vi "niRFUtil CONV 1 Ohm Voltage to dBm (complex scalar).vi"(7 "Complex Scalar (V)":csg format="%.2f") -> (8 "Real Scalar (dBm)":sgl format="%.2f")   [LabVIEW 2015, in "niRFUtil.lvlib"]
doc: "(c) Copyright 2006, National Instruments, Inc. This VI may not be duplicated, sold, or distributed without written consent from National Instruments."
uses:
  niRFUtil.lvlib
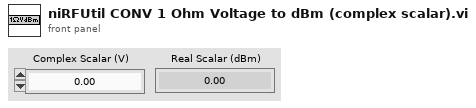
[diagram p1: front panel]
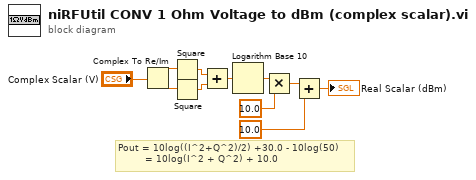
[diagram p0: block diagram]
diagram:
  # "Pout = 10log((I^2+Q^2)/2) +30.0 - 10log(50)\n         = 10log(I^2 + Q^2) + 10.0"
  n1 = Complex To Re/Im(x + iy="Complex Scalar (V)") -> (x=w7:sgl, y=w6:sgl)
  n2 = Square(x=w7) -> (x^2=w5:sgl)
  n3 = Square(x=w6) -> (x^2=w4:sgl)
  n4 = Add(x=w5, y=w4) -> (x+y=w3:sgl)
  n5 = Logarithm Base 10(1:w3) -> (0:w11:sgl)
  n6 = Multiply(x=w11, y=sgl 10.0) -> (x*y=w9:sgl)
  n7 = Add(x=w9, y=sgl 10.0) -> (x+y=→"Real Scalar (dBm)":sgl)
